vi "input.vi"() -> ()   [LabVIEW 2015]
doc: "This vi receives udp packets from labview and converts them from string to the appropriate data types and are then stored in a cluster."
uses:
  global.vi
panel:
  out "String":string
  out "FG Data":T1
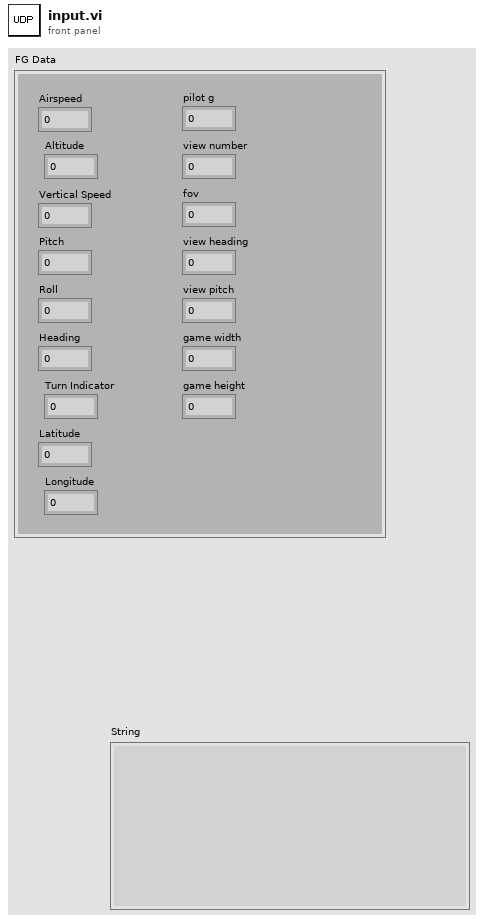
[diagram p1: front panel]
types:
  T1 = cluster{"Airspeed":dbl, "Altitude":dbl, "Vertical Speed":dbl, "Pitch":dbl, "Roll":dbl, "Heading":dbl, "Turn Indicator":dbl, "Latitude":dbl, "Longitude":dbl, "pilot g":dbl, "view number":i16, "fov":dbl, "view heading":dbl, "view pitch":dbl, "game width":i16, "game height":i16}
  T2 = cluster{dbl, dbl, dbl, dbl, dbl, dbl, dbl, dbl, dbl, dbl, i16, dbl, dbl, dbl, i16, i16}
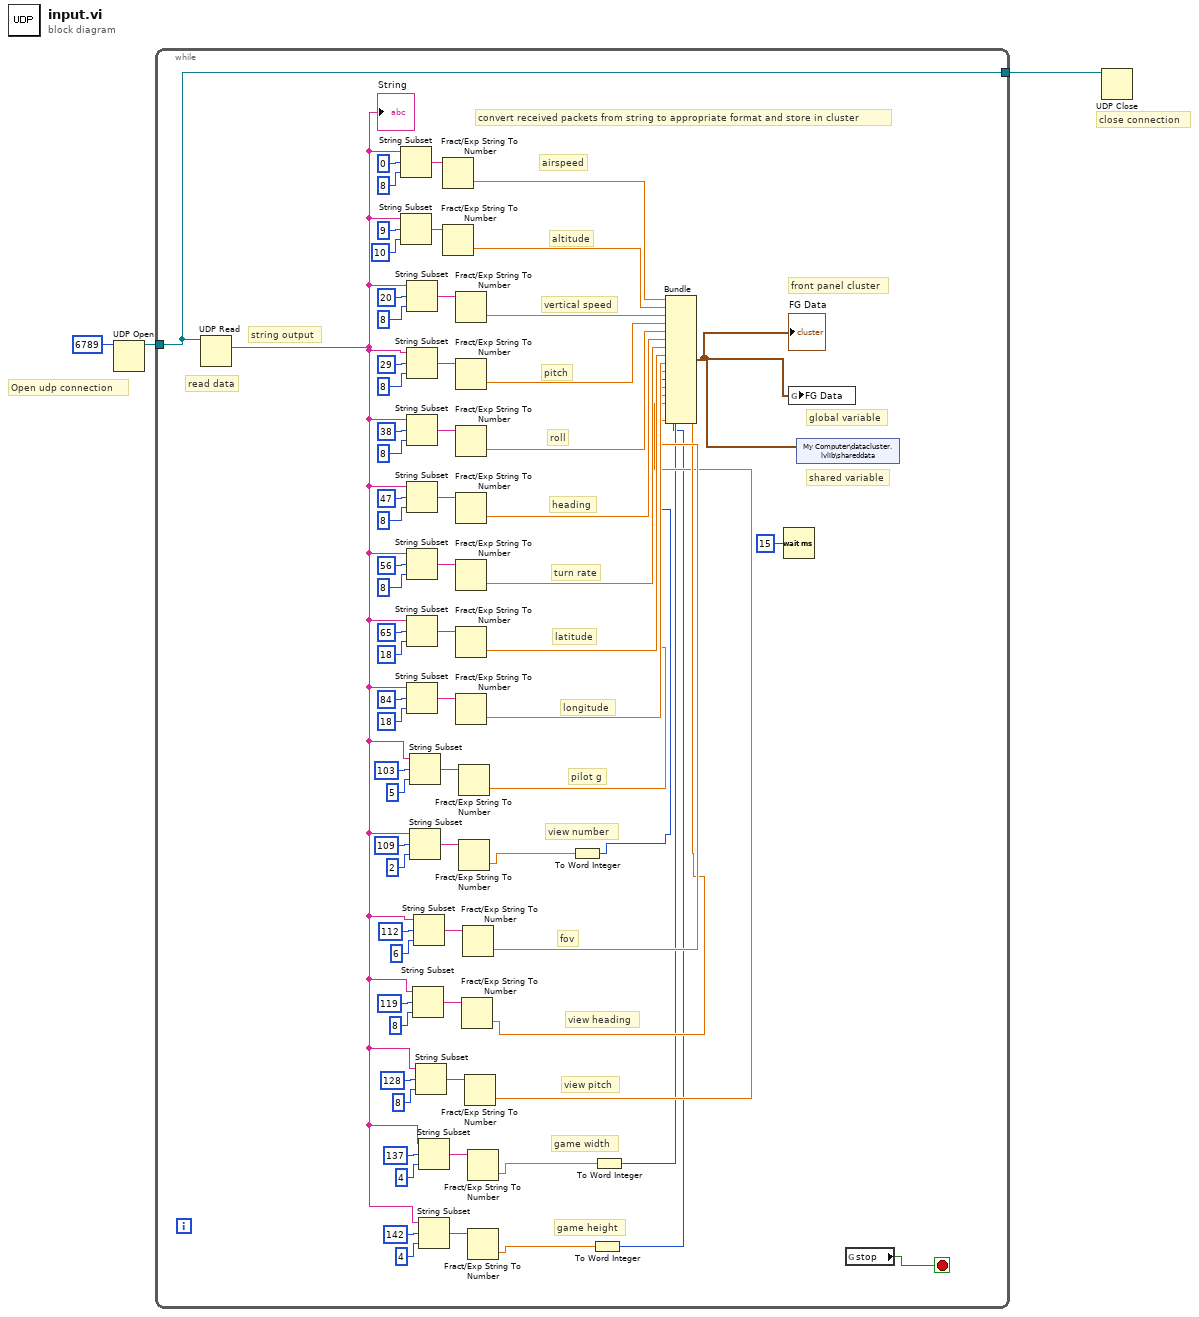
[diagram p0: block diagram]
diagram:
  # "close connection"
  # "Open udp connection"
  n1 = UDP Open(11:u16 6789 ("port")) -> (port=w2:refnum<k16>)  [unwired: 4 in, 2 out]
  n2 = while {
    tunnel: w2 -> [w40]
    tunnel: [w40] -> w1
    stop <- w4 stop-if-true
    # "front panel cluster"
    # "global variable"
    # "shared variable"
    # "string output"
    # "read data"
    # "game height"
    # "game width"
    # "view pitch"
    # "view heading"
    # "fov"
    # "view number"
    # "pilot g"
    # "convert received packets from string to appropriate format and store in cluster"
    # "longitude"
    # "latitude"
    # "turn rate"
    # "heading"
    # "roll"
    # "pitch"
    # "vertical speed"
    # "altitude"
    # "airspeed"
    n3 = UDP Read(connection ID=w40) -> (data out=w17:string)  [unwired: 3 in, 4 out]
    "String" <- w17
    n4 = String Subset(string=w17, offset (0)=0, length (rest)=8 ("length (rest)")) -> (substring=w41:string)
    n5 = String Subset(string=w17, offset (0)=9, length (rest)=10 ("length (rest)")) -> (substring=w5:string)
    n6 = String Subset(string=w17, offset (0)=20, length (rest)=8 ("length (rest)")) -> (substring=w69:string)
    n7 = String Subset(string=w17, offset (0)=29, length (rest)=8 ("length (rest)")) -> (substring=w68:string)
    n8 = String Subset(string=w17, offset (0)=38, length (rest)=8 ("length (rest)")) -> (substring=w67:string)
    n9 = String Subset(string=w17, offset (0)=47, length (rest)=8 ("length (rest)")) -> (substring=w66:string)
    n10 = String Subset(string=w17, offset (0)=56, length (rest)=8 ("length (rest)")) -> (substring=w65:string)
    n11 = String Subset(string=w17, offset (0)=65, length (rest)=18 ("length (rest)")) -> (substring=w64:string)
    n12 = String Subset(string=w17, offset (0)=84, length (rest)=18 ("length (rest)")) -> (substring=w63:string)
    n13 = String Subset(string=w17, offset (0)=103, length (rest)=5 ("length (rest)")) -> (substring=w38:string)
    n14 = String Subset(string=w17, offset (0)=109, length (rest)=2 ("length (rest)")) -> (substring=w35:string)
    n15 = String Subset(string=w17, offset (0)=119, length (rest)=8 ("length (rest)")) -> (substring=w29:string)
    n16 = String Subset(string=w17, offset (0)=112, length (rest)=6 ("length (rest)")) -> (substring=w32:string)
    n17 = String Subset(string=w17, offset (0)=128, length (rest)=8 ("length (rest)")) -> (substring=w26:string)
    n18 = String Subset(string=w17, offset (0)=137, length (rest)=4 ("length (rest)")) -> (substring=w23:string)
    n19 = String Subset(string=w17, offset (0)=142, length (rest)=4 ("length (rest)")) -> (substring=w20:string)
    n20 = Fract/Exp String To Number(string=w41) -> (number=w71:dbl)  [unwired: 3 in, 1 out]
    n21 = Fract/Exp String To Number(string=w5) -> (number=w70:dbl)  [unwired: 3 in, 1 out]
    n22 = Fract/Exp String To Number(string=w69) -> (number=w62:dbl)  [unwired: 3 in, 1 out]
    n23 = Fract/Exp String To Number(string=w68) -> (number=w61:dbl)  [unwired: 3 in, 1 out]
    n24 = Fract/Exp String To Number(string=w67) -> (number=w60:dbl)  [unwired: 3 in, 1 out]
    n25 = Fract/Exp String To Number(string=w66) -> (number=w59:dbl)  [unwired: 3 in, 1 out]
    n26 = Fract/Exp String To Number(string=w65) -> (number=w58:dbl)  [unwired: 3 in, 1 out]
    n27 = Fract/Exp String To Number(string=w64) -> (number=w57:dbl)  [unwired: 3 in, 1 out]
    n28 = Fract/Exp String To Number(string=w63) -> (number=w56:dbl)  [unwired: 3 in, 1 out]
    n29 = Fract/Exp String To Number(string=w38) -> (number=w13:dbl)  [unwired: 3 in, 1 out]
    n30 = Fract/Exp String To Number(string=w35) -> (number=w14:dbl)  [unwired: 3 in, 1 out]
    n31 = Fract/Exp String To Number(string=w29) -> (number=w10:dbl)  [unwired: 3 in, 1 out]
    n32 = Fract/Exp String To Number(string=w32) -> (number=w11:dbl)  [unwired: 3 in, 1 out]
    n33 = Fract/Exp String To Number(string=w26) -> (number=w9:dbl)  [unwired: 3 in, 1 out]
    n34 = Fract/Exp String To Number(string=w23) -> (number=w15:dbl)  [unwired: 3 in, 1 out]
    n35 = Fract/Exp String To Number(string=w20) -> (number=w16:dbl)  [unwired: 3 in, 1 out]
    n36 = To Word Integer(number=w14) -> (16bit integer=w12:i16)
    n37 = To Word Integer(number=w16) -> (16bit integer=w7:i16)
    n38 = To Word Integer(number=w15) -> (16bit integer=w8:i16)
    n39 = Bundle(w71, w70, w62, w61, w60, w59, w58, w57, w56, w13, w12, w11, w10, w9, w8, w7) -> (w6:T2)  [unwired: 1 in]
    "FG Data" <- w6
    n40 = Wait (ms)(milliseconds to wait=u32 15) -> ()  [unwired: 1 out]
    n41 = global write "global.vi" "FG Data"(w6) -> ()
    n42 = shared-variable "My Computer\\datacluster.lvlib\\shareddata"(w6) -> ()  [unwired: 1 in, 1 out]
    n43 = global read "global.vi" "stop"() -> (w4:bool)
  }
  n44 = UDP Close(connection ID=w1) -> ()  [unwired: 1 in, 2 out]
